vi "质控模块润洗OK命令.vi"(8 "error in (no error)":errorcluster, 11 "质控润洗OK":bool) -> (0 "error out":errorcluster)   [LabVIEW 2016, in "质控单元V4.lvlib"]
uses:
  <vilib>/Plasmionique/MB Master/MB Master.lvlib
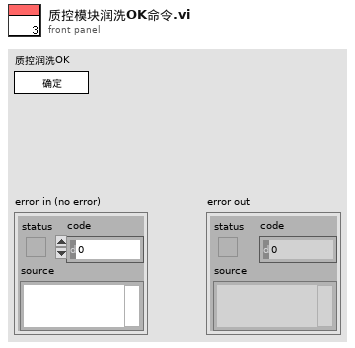
[diagram p1: front panel]
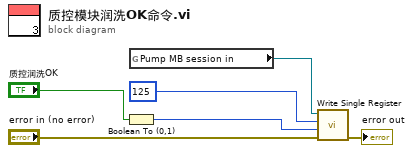
[diagram p0: block diagram]
diagram:
  n1 = Boolean To (0,1)(Boolean="质控润洗OK") -> (0, 1=w1:i16)
  n2 = global read "系统交互.vi" "Pump MB session in"() -> (w4:refnum<class "MB_Master.lvclass">)
  n3 = call <vilib>:"Write Single Register.vi"("error in (no error)"="error in (no error)", "value"=w1, "address"=u16 125 ("starting address"), "MB session in"=w4) -> ("error out"=→"error out":errorcluster)  [unwired: 6 in, 1 out]
